vi "Get Targets_Do.vi"(8 "error in (no error)":errorcluster, 11 "Dependency Source_NIPM in":refnum<class "Dependency Source_GPM.lvclass">) -> (0 "error out":errorcluster, 1 "Success?":bool, 2 "External Target Map":map{string, string}(c390), 3 "Internal Target Map":map{string, string}(c390), 4 "Unhandled Targets":string[](array[string]))   [LabVIEW 2019, in "Project.Dependencies Finder.lvlib" / "Dependency Source_GPM.lvclass"]
doc: "Get targets for the dependency source (GPM is mostly external).\n\nLoads GPM_External.txt and GPM_Internal.txt and returns the results. \n\nGPM_External.txt contains only the package name [author]/[Package name].\nGPM_Internal.txt contains data in the following format: [package name][tab][path1]:[path2]:...\n\nNote: the method of this class will be changed when a better way to find the package paths is found."
uses:
  Dependency Source_GPM.lvclass
  f60522bd-8f4c-4ca2-88d6-941245162926.vi
  <vilib>/Utility/file.llb/Read Delimited Spreadsheet (string).vi
  Project.Dependencies Finder.lvlib
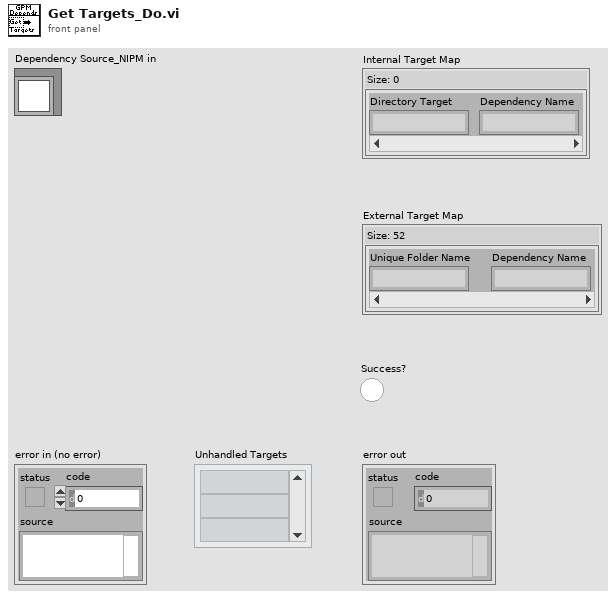
[diagram p1: front panel]
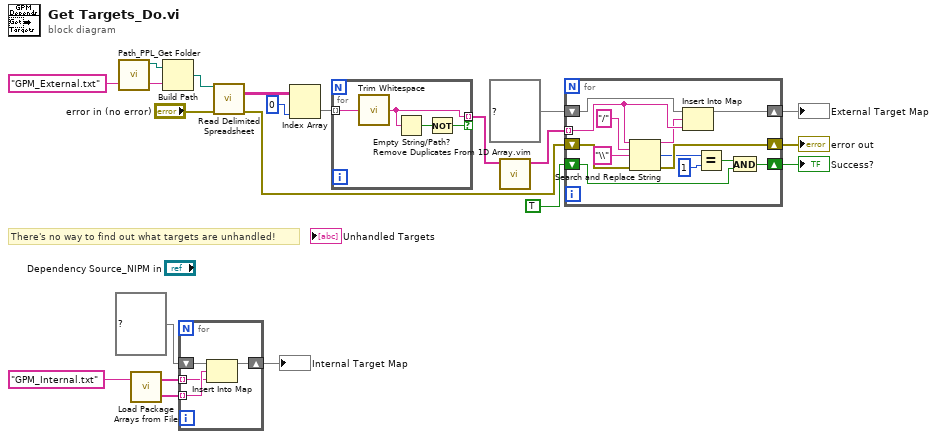
[diagram p0: block diagram]
diagram:
  # "There's no way to find out what targets are unhandled!"
  n1 = call <userlib>:"Path_PPL_Get Folder.vi"() -> ("PPL Folder Path (from PPL)"=w19:path)  [unwired: 11 in]
  n2 = call "Load Package Arrays from File.vi"("File name"="GPM_Internal.txt" ("name or relative path")) -> ("Path Identifier Array"=w2:string[], "Package Name Array"=w1:string[])  [unwired: 1 in]
  n3 = Build Path(base path=w19, name or relative path="GPM_External.txt") -> (appended path=w16:path)
  n4 = for {
    shift-right: [w23] -> w3
    shift-left: map{string, string} {} ("Internal Target Map") -> [w24]
    tunnel: w2 -> [w22] mode=indexing
    tunnel: w1 -> [w21] mode=indexing
    n5 = Insert Into Map(map in=w24, key=w22, value=w21) -> (map out=w23:map{string, string})  [unwired: 2 out]
  }
  "Internal Target Map" <- w3
  n6 = call-poly <vilib>:"Read Delimited Spreadsheet.vi"("file path (dialog if empty)"=w16, "error in (no error)"="error in (no error)") -> ("all rows"=w15:string[][], "error out"=w11:errorcluster)  [unwired: 8 in, 4 out]
  n7 = Index Array(array=w15, index (col)=0 ("disabled index (col)")) -> (element=w7:string[])  [unwired: 1 in]
  n8 = for {
    tunnel: w7 -> [w28] mode=indexing
    tunnel: [w26] -> w6 mode=indexing if=w25
    n9 = call <vilib>:"Trim Whitespace.vi"("string"=w28) -> ("trimmed string"=w26:string)  [unwired: 1 in]
    n10 = Empty String/Path?(string/path=w26) -> (empty?=w27:bool)
    n11 = Not(x=w27) -> (.not. x?=w25:bool)
  }
  n12 = call "Remove Duplicates From 1D Array.vim"("array"=w6) -> ("array with duplicates removed"=w12:string[])  [unwired: 10 in]
  n13 = for {
    shift-right: [w40] -> w17
    shift-left: map{string, string} {} ("External Target Map") -> [w41]
    tunnel: w12 -> [w39] mode=indexing
    shift-right: [w34] -> w10
    shift-left: w11 -> [w35]
    shift-right: [w29] -> w8
    shift-left: TRUE -> [w30]
    n14 = Search and Replace String(input string=w39, search string="/", replace string="\\" ("replace string (\"\")"), error in=w35) -> (result string=w36:string, number of replacements=w33:i32, error out=w34:errorcluster)  [unwired: 4 in, 1 out]
    n15 = Insert Into Map(map in=w41, key=w36, value=w39) -> (map out=w40:map{string, string})  [unwired: 2 out]
    n16 = Equal?(x=w33, y=1) -> (x = y?=w31:bool)
    n17 = And(x=w31, y=w30) -> (x .and. y?=w29:bool)
  }
  "error out" <- w10
  "Success?" <- w8
  "External Target Map" <- w17
